vi "vonKarmanFit.vi"(6 "lambdaEstimate":dbl=1.0, 7 "MaxFitFreq":dbl, 9 "U(h)":dbl, 10 "f.E(f)":dbl[](array[numeric]), 11 "f":dbl[](array[numeric])) -> (0 "lambda":dbl format="%#_4g", 1 "vonKarmanFitEquation":string, 2 "CroppedData":cluster{"X Out":dbl[], "Y Out":dbl[]}, 3 "FitCurve":T1, 4 "a":dbl format="%#_4g")   [LabVIEW 2016]
uses:
  <vilib>/Analysis/6fits.llb/Remove Outliers (Range).vi
  <vilib>/gmath/NumericalOptimization/Nonlinear Curve Fit LM formula string.vi
  <vilib>/gmath/NI_Gmath.lvlib
  <vilib>/Analysis/NI_AALPro.lvlib
panel:
  out "vK integral":dbl
  out "Band-limited Integral":dbl
  out "FullSpectrumIntegral":dbl
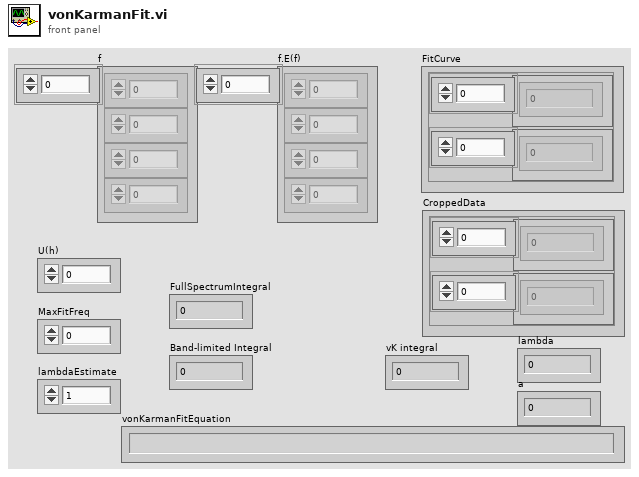
[diagram p1: front panel]
types:
  T1 = cluster{"Array":dbl[], "best nonlinear fit":dbl[]}
  T2 = cluster{"model":string, "Parameters":string[], "x":string}
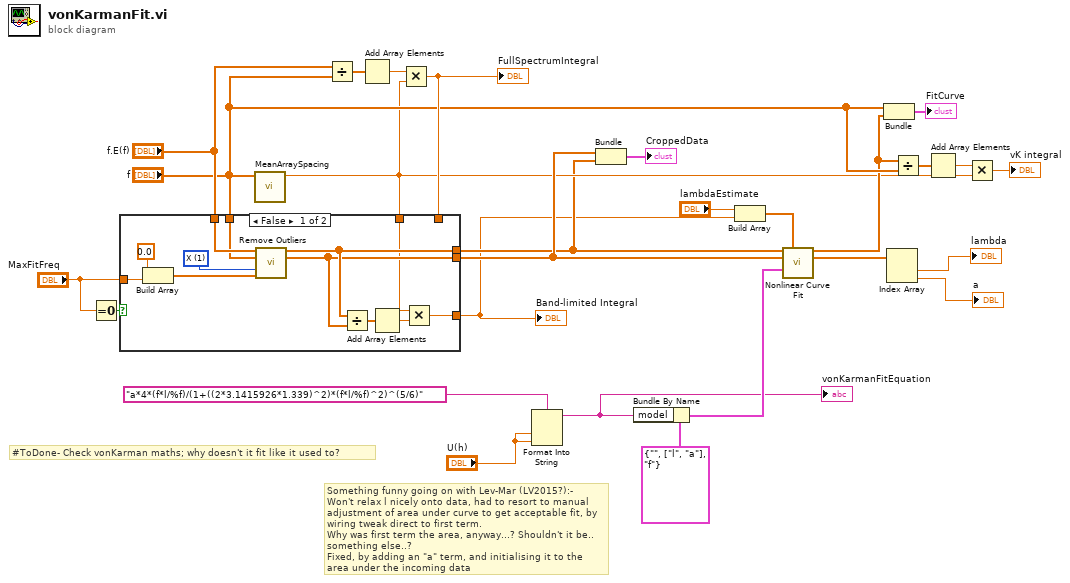
[diagram p0: block diagram]
diagram:
  # "#ToDone- Check vonKarman maths; why doesn't it fit like it used to?"
  # "Something funny going on with Lev-Mar (LV2015?):-\nWon't relax l nicely onto data, had to resort to manual adjustment of area under curve to get acceptable fit, by wiring tweak direct to first term.\nWhy was first term the area, anyway...? Shouldn't it be.. something else..?\nFixed, by adding an \"a\" term, and initialising it to the area under the incoming data"
  n1 = Equal To 0?(x="MaxFitFreq") -> (x = 0?=w12:bool)
  n2 = call "MeanArraySpacing.vi"("Array"="f") -> ("Mean Spacing"=w5:dbl)  [unwired: 10 in]
  n3 = Divide(x="f.E(f)", y="f") -> (x/y=w18:dbl[])
  n4 = Add Array Elements(numeric array=w18) -> (sum=w19:dbl)
  n5 = Multiply(x=w19, y=w5) -> (x*y=w10:dbl)
  "FullSpectrumIntegral" <- w10
  n6 = case shown="False" w12 {
    tunnel: [w39 w41] -> w3
    tunnel: [w38 w42] -> w27
    tunnel: [w36 w40] -> w2
    tunnel: "f.E(f)" -> [w33 w41]
    tunnel: "f" -> [w31 w42]
    tunnel: "MaxFitFreq" -> [w29 _]
    tunnel: w5 -> [w28 _]
    tunnel: w10 -> [_ w40]
    frame False {
      w34 = u16 1 items=["x", "X", "X and Y"] ("range type")
      n7 = Build Array(0.0 ("element"), w29) -> (w30:dbl[])
      n8 = call-poly <vilib>:"Remove Outliers.vi"("Y"=w33, "X"=w31, "range type"=w34, "Range"=w30) -> ("Y Out"=w39:dbl[], "X Out"=w38:dbl[])  [unwired: 7 in, 3 out]
      n9 = Divide(x=w39, y=w38) -> (x/y=w37:dbl[])
      n10 = Add Array Elements(numeric array=w37) -> (sum=w35:dbl)
      n11 = Multiply(x=w28, y=w35) -> (x*y=w36:dbl)
    }
    frame True {
    }
  }
  "Band-limited Integral" <- w2
  n12 = Format Into String(format string="a*4*(f*l/%f)/(1+((2*3.1415926*1.339)^2)*(f*l/%f)^2)^(5/6)" ("vonKarman Spectrum"), "U(h)", "U(h)") -> (resulting string=w11:string)  [unwired: 2 in, 1 out]
  "vonKarmanFitEquation" <- w11
  n13 = Bundle("f"=w27, "f.E(f)"=w3) -> (→"CroppedData":cluster{"f":dbl[], "f.E(f)":dbl[]})  [unwired: 1 in]
  n14 = Bundle By Name(cluster=T2 {"model"="", "Parameters"=["l", "a"], "x"="f"} ("model description"), "model"=w11) -> (w22:T2)
  n15 = Build Array("lambdaEstimate", w2) -> (w16:dbl[])
  n16 = call-poly <vilib>:"Nonlinear Curve Fit.vi"("Y"=w3, "initial parameters"=w16, "X"=w27, "model description"=w22) -> ("best nonlinear fit"=w6:dbl[], "best fit parameters"=w20:dbl[])  [unwired: 7 in, 3 out]
  n17 = Bundle("f"="f", "best nonlinear fit"=w6) -> (→"FitCurve":cluster{"f":dbl[], "best nonlinear fit":dbl[]})  [unwired: 1 in]
  n18 = Index Array(array=w20) -> (element #1=→"lambda":dbl, element #2=→"a":dbl)  [unwired: 2 in]
  n19 = Divide(x=w6, y="f") -> (x/y=w9:dbl[])
  n20 = Add Array Elements(numeric array=w9) -> (sum=w8:dbl)
  n21 = Multiply(x=w8, y=w5) -> (x*y=→"vK integral":dbl)
